vi "FFTBoost.vi"(7 "CompensationCoefficients":dbl[](array[numeric])=[1.0, 1.0, 0.0, 0.0, 0.0], 9 "PhaseCorrection":dbl[](array[numeric]), 10 "mutedData":dbl[](array[numeric])=array[1605632 elements]) -> (2 "boostedData":dbl[](array[numeric]))   [LabVIEW 2012]
uses:
  <vilib>/Analysis/2dsp.llb/Real FFT.vi
  <vilib>/Analysis/2dsp.llb/Inverse Real FFT.vi
  <vilib>/Analysis/NI_AALPro.lvlib
panel:
  out "CallCount":dbl
  out "Waveform Graph":cluster{i32, i32, dbl[]}[](graph)
  # "NOTE- This VI DOES NOT preserve means- they should be calculated before, and re-added after, compensation"
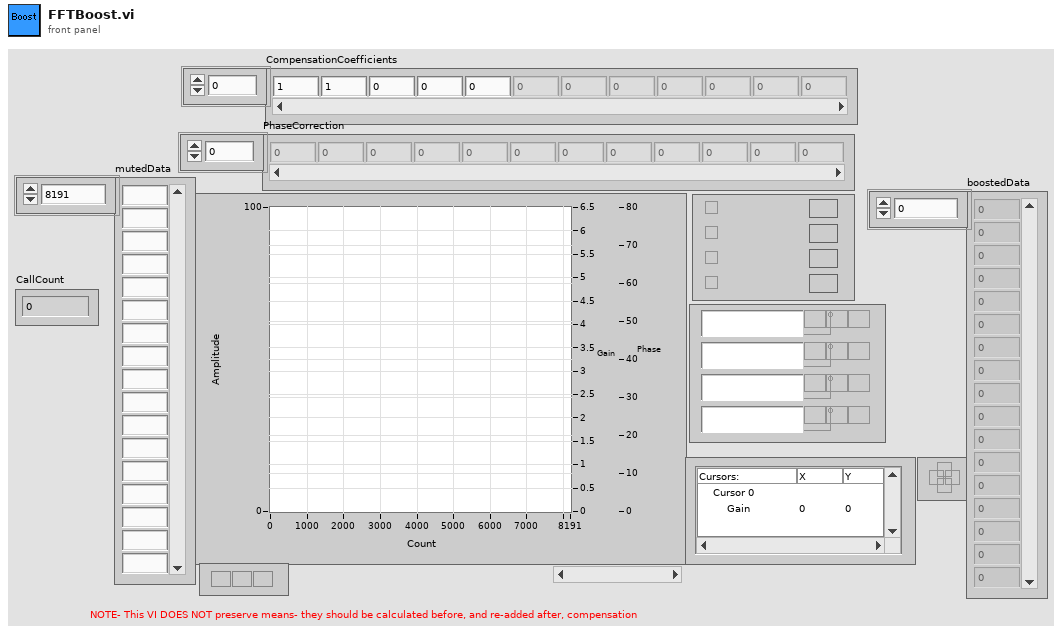
[diagram p1: front panel]
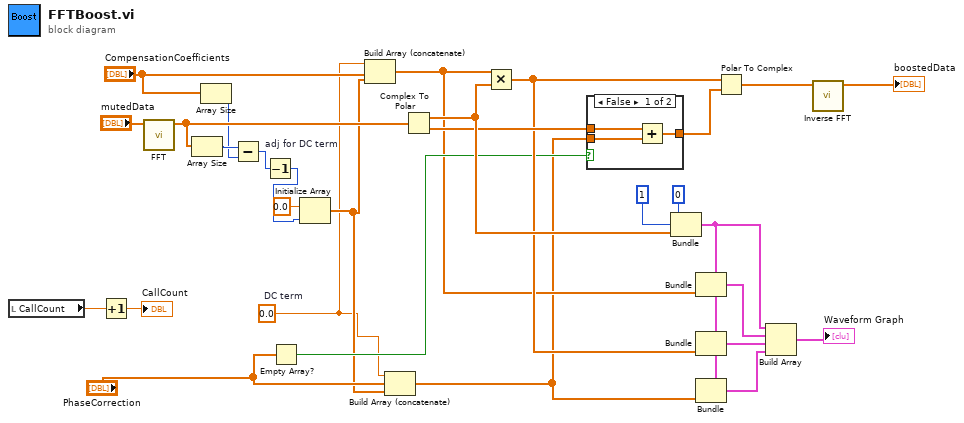
[diagram p0: block diagram]
diagram:
  w1 = 0.0  # DC term
  n1 = local read "CallCount"() -> (w23:dbl)
  n2 = Increment(x=w23) -> (x+1=→"CallCount":dbl)
  n3 = call-poly <vilib>:"FFT.vi"("X"="mutedData") -> ("FFT {X}"=w11:cdb[])  [unwired: 2 in, 8 out]
  n4 = Array Size(array=w11) -> (size(s)=w10:i32)
  n5 = Array Size(array="CompensationCoefficients") -> (size(s)=w9:i32)
  n6 = Subtract(x=w10, y=w9) -> (x-y=w8:i32)
  n7 = Decrement "adj for DC term"(x=w8) -> (x-1=w2:i32)
  n8 = Empty Array?(array="PhaseCorrection") -> (empty?=w16:bool)
  n9 = Initialize Array(0.0 ("element"), w2) -> (w3:dbl[])
  n10 = Build Array (concatenate)(w1, "CompensationCoefficients", w3) -> (w7:dbl[])
  n11 = Build Array (concatenate)(w1, "PhaseCorrection", w3) -> (w4:dbl[])
  n12 = Complex To Polar(r * e^(i*theta)=w11) -> (r=w21:dbl[], theta=w20:dbl[])
  n13 = Multiply(x=w7, y=w21) -> (x*y=w18:dbl[])
  n14 = case shown="False" w16 {
    tunnel: w4 -> [w30 _]
    tunnel: w20 -> [w31 w33]
    tunnel: [w32 w33] -> w19
    frame False {
      n15 = Add(x=w31, y=w30) -> (x+y=w32:dbl[])
    }
    frame True {
    }
  }
  n16 = Bundle(0, 1, w21) -> (w14:cluster{i32, i32, dbl[]})  [unwired: 1 in]
  n17 = Bundle(cluster=w14, w7) -> (w28:cluster{i32, i32, dbl[]})  [unwired: 2 in]
  n18 = Bundle(cluster=w14, w18) -> (w27:cluster{i32, i32, dbl[]})  [unwired: 2 in]
  n19 = Bundle(cluster=w14, w4) -> (w13:cluster{i32, i32, dbl[]})  [unwired: 2 in]
  n20 = Polar To Complex(1:w19, 2:w18) -> (0:w17:cdb[])
  n21 = Build Array(w14, w28, w27, w13) -> (→"Waveform Graph":cluster{i32, i32, dbl[]}[])
  n22 = call-poly <vilib>:"Inverse FFT.vi"("FFT {X}"=w17) -> ("X"=→"boostedData":dbl[])  [unwired: 1 in, 9 out]
